vi "DAQgates_init.vi"() -> ()   [LabVIEW 2012]
uses:
  <vilib>/DAQmx/write.llb/DAQmx Write (Analog 1D DBL NChan 1Samp).vi
  <vilib>/DAQmx/read.llb/DAQmx Read (Analog 1D DBL NChan 1Samp).vi
  <vilib>/DAQmx/create/channels.llb/DAQmx Create Channel (AO-Voltage-Basic).vi
  <vilib>/DAQmx/miscellaneous.llb/DAQmx Fill In Error Info.vi
  <vilib>/DAQmx/create/channels.llb/DAQmx Create Channel (AI-Voltage-Basic).vi
panel:
  in  "Static Channels 2":cluster{dbl, string, "Output Channels":tag}[](array[cluster])=[{1.0, "", "Output Channels"="Dev1/ao2"}, {1.0, "", "Output Channels"="Dev1/ao3"}, {1.0, "", "Output Channels"="Dev2/ao2"}, {1.0, "", "Output Channels"="Dev2/ao3"}, {0.0, "", "Output Channels"=""}, {1.0, "", "Output Channels"=""}]
  out "error out":errorcluster
  out "data":dbl[](array[numeric]) format="%0.2f"
  in  "Output 2":dbl step=0.05
  in  "Output 1":dbl step=0.03
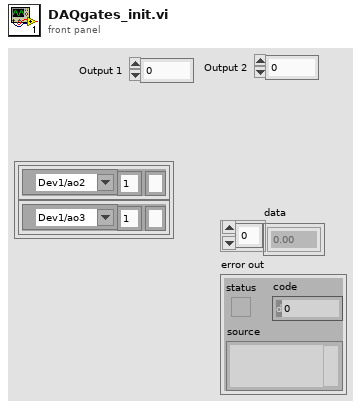
[diagram p1: front panel]
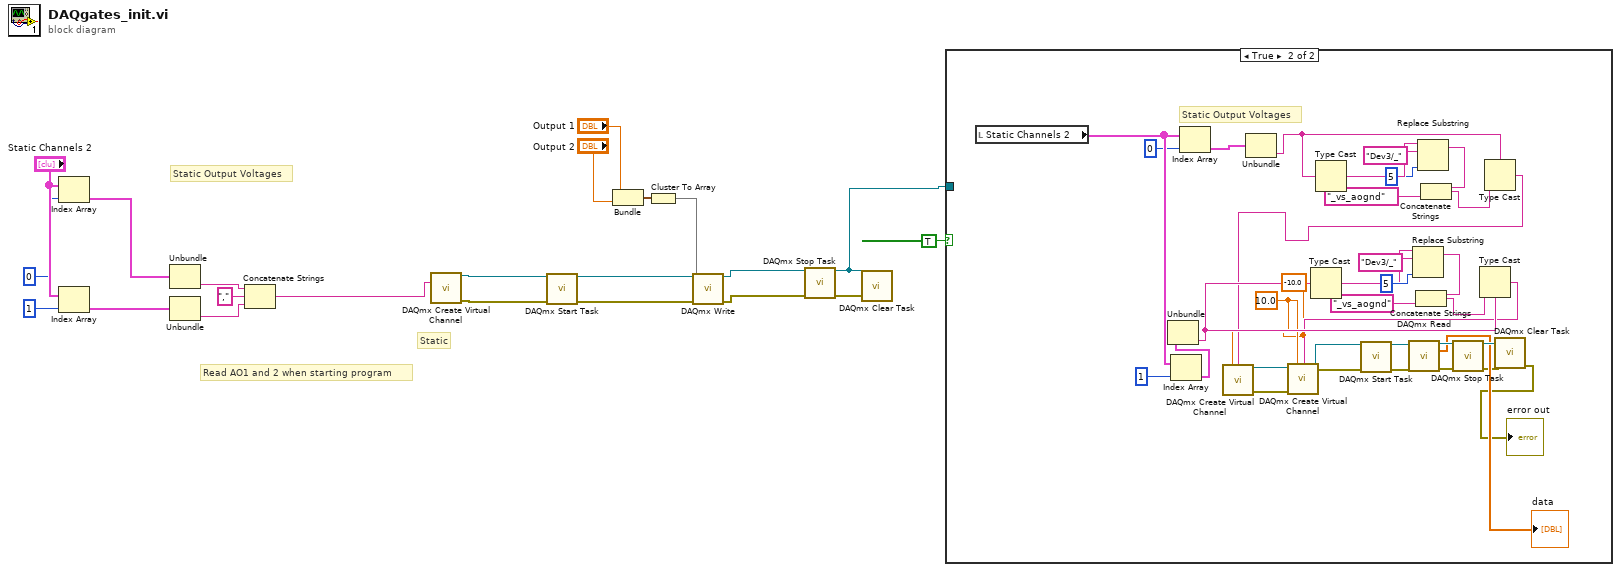
[diagram p0: block diagram]
diagram:
  # "Static Output Voltages"
  # "Static"
  # "Read AO1 and 2 when starting program"
  n1 = Index Array(array="Static Channels 2", index=0) -> (element=w6:cluster{dbl, string, "Output Channels":tag})
  n2 = Index Array(array="Static Channels 2", index=1) -> (element=w7:cluster{dbl, string, "Output Channels":tag})
  n3 = Unbundle(w6) -> ("Output Channels"=w12:tag)  [unwired: 2 out]
  n4 = Unbundle(w7) -> ("Output Channels"=w11:tag)  [unwired: 2 out]
  n5 = Concatenate Strings(w12, ",", w11) -> (w5:string)
  n6 = call-poly <vilib>:"DAQmx Create Virtual Channel.vi"("physical channels"=w5) -> ("task out"=w17:refnum<k21>, "error out"=w16:errorcluster)  [unwired: 13 in]
  n7 = call <vilib>:"DAQmx Start Task.vi"("task/channels in"=w17, "error in"=w16) -> ("task out"=w15:refnum<k21>, "error out"=w14:errorcluster)  [unwired: 12 in]
  n8 = Bundle("Output 1"="Output 1", "Output 2"="Output 2") -> (w21:cluster{"Output 1":dbl, "Output 2":dbl})  [unwired: 1 in]
  n9 = Cluster To Array(cluster=w21) -> (array=w20:dbl[])
  n10 = call-poly <vilib>:"DAQmx Write.vi"("task/channels in"=w15, "data"=w20, "error in"=w14) -> ("task out"=w4:refnum<k21>, "error out"=w3:errorcluster)  [unwired: 10 in, 1 out]
  n11 = call <vilib>:"DAQmx Stop Task.vi"("task/channels in"=w4, "error in"=w3) -> ("task out"=w1:refnum<k21>, "error out"=w2:errorcluster)  [unwired: 12 in]
  n12 = call <vilib>:"DAQmx Clear Task.vi"("task in"=w1, "error in"=w2) -> ()  [unwired: 13 in, 1 out]
  n13 = case shown="True" TRUE {
    tunnel: w1 -> [_ _]
    frame False {
    }
    frame True {
      w27 = -10.0 ("minimum value")
      w28 = 10.0 ("maximum value")
      # "Static Output Voltages"
      n14 = local read "Static Channels 2"() -> (w57:cluster{dbl, string, "Output Channels":tag}[])
      n15 = Index Array(array=w57, index=1) -> (element=w55:cluster{dbl, string, "Output Channels":tag})
      n16 = Unbundle(w55) -> ("Output Channels"=w44:tag)  [unwired: 2 out]
      n17 = Index Array(array=w57, index=0) -> (element=w56:cluster{dbl, string, "Output Channels":tag})
      n18 = Unbundle(w56) -> ("Output Channels"=w37:tag)  [unwired: 2 out]
      n19 = Type Cast(x=w44) -> (*(type *) &x=w47:string)  [unwired: 1 in]
      n20 = Type Cast(x=w37) -> (*(type *) &x=w43:string)  [unwired: 1 in]
      n21 = Replace Substring(2:5 ("length (len. of substring)"), 4:"Dev3/_" ("substring (\"\")"), 5:w47) -> (1:w50:string)  [unwired: 1 in, 1 out]
      n22 = Concatenate Strings(w50, "_vs_aognd" ("string")) -> (w52:string)
      n23 = Replace Substring(2:5 ("length (len. of substring)"), 4:"Dev3/_" ("substring (\"\")"), 5:w43) -> (1:w40:string)  [unwired: 1 in, 1 out]
      n24 = Concatenate Strings(w40, "_vs_aognd" ("string")) -> (w38:string)
      n25 = Type Cast(type=w44, x=w52) -> (*(type *) &x=w34:tag)
      n26 = Type Cast(type=w37, x=w38) -> (*(type *) &x=w36:tag)
      n27 = call-poly <vilib>:"DAQmx Create Virtual Channel.vi"("maximum value"=w28, "minimum value"=w27, "physical channels"=w36) -> ("task out"=w35:refnum<k21>, "error out"=w29:errorcluster)  [unwired: 11 in]
      n28 = call-poly <vilib>:"DAQmx Create Virtual Channel.vi"("task in"=w35, "maximum value"=w28, "minimum value"=w27, "physical channels"=w34, "error in"=w29) -> ("task out"=w24:refnum<k21>, "error out"=w23:errorcluster)  [unwired: 9 in]
      n29 = call <vilib>:"DAQmx Start Task.vi"("task/channels in"=w24, "error in"=w23) -> ("task out"=w26:refnum<k21>, "error out"=w25:errorcluster)  [unwired: 12 in]
      n30 = call-poly <vilib>:"DAQmx Read.vi"("task/channels in"=w26, "error in"=w25) -> ("task out"=w45:refnum<k21>, "data"=→"data":dbl[], "error out"=w30:errorcluster)  [unwired: 11 in]
      n31 = call <vilib>:"DAQmx Stop Task.vi"("task/channels in"=w45, "error in"=w30) -> ("task out"=w46:refnum<k21>, "error out"=w31:errorcluster)  [unwired: 12 in]
      n32 = call <vilib>:"DAQmx Clear Task.vi"("task in"=w46, "error in"=w31) -> ("error out"=→"error out":errorcluster)  [unwired: 13 in]
    }
  }
